vi "sub vi - GET ALL TEMP v6.vi"(0 "LA01-EN":bool, 1 "simulate":bool, 5 "LA02-EN":bool, 7 "LA03-EN":bool, 9 "LA04-EN":bool, 11 "LA05-EN":bool, 12 "Gen Cal Value":dbl) -> (4 "LA01 TEMP":T1, 6 "LA02 TEMP":T1, 8 "LA03 TEMP":T1, 10 "LA04 TEMP":T1, 14 "error":bool, 15 "LA05 TEMP":T1)   [LabVIEW 2013]
uses:
  program files/Global display 4.vi
panel:
  out "LOOP TIME":dbl
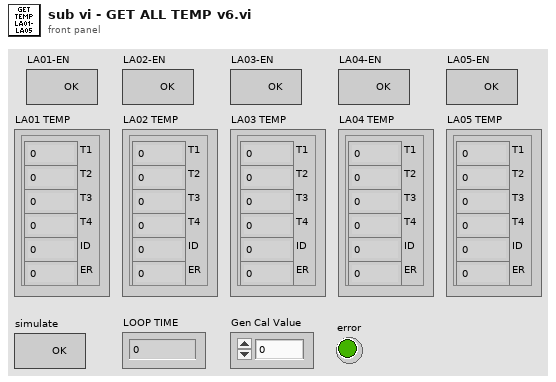
[diagram p1: front panel]
types:
  T1 = cluster{"T1":dbl, "T2":dbl, "T3":dbl, "T4":dbl, "ID":dbl, "ER":dbl}
  T2 = cluster{"1 TL":dbl, "1 TN":dbl, "2 TL":dbl, "2 TN":dbl, "ID":dbl, "ER":dbl}
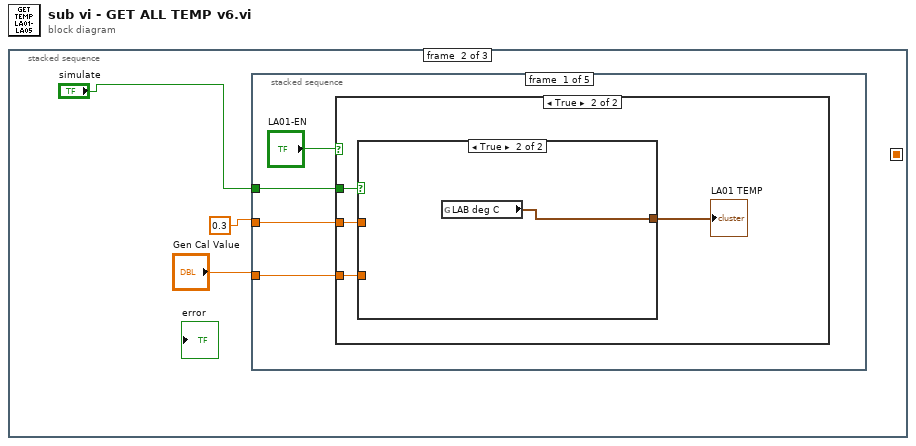
[diagram p0: block diagram]
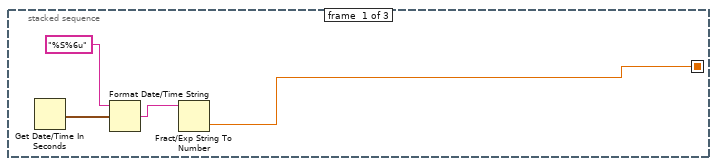
[diagram p2: hidden frame]
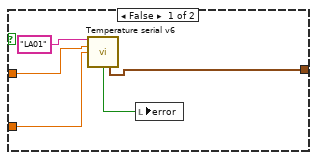
[diagram p4: hidden frame]
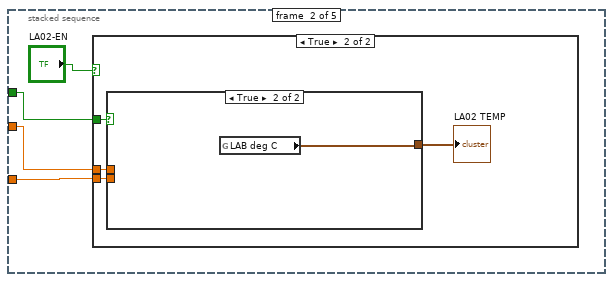
[diagram p5: hidden frame]
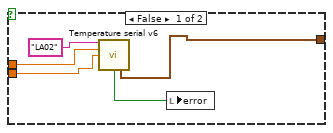
[diagram p7: hidden frame]
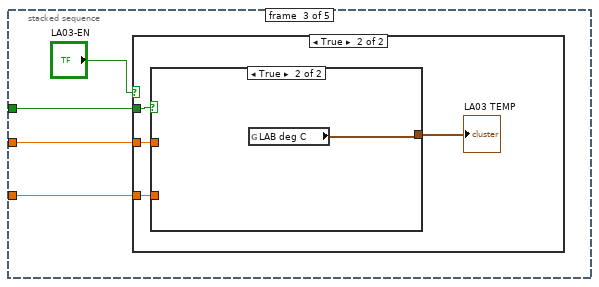
[diagram p8: hidden frame]
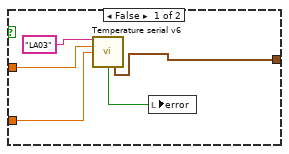
[diagram p10: hidden frame]
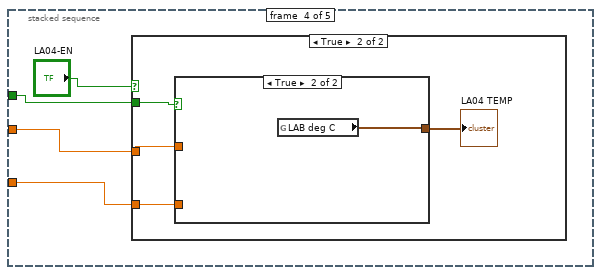
[diagram p11: hidden frame]
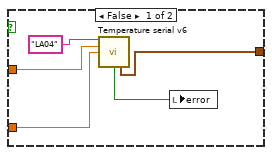
[diagram p13: hidden frame]
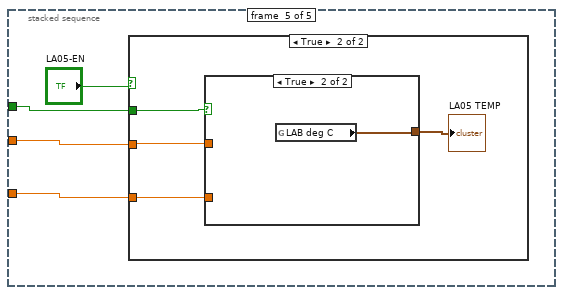
[diagram p14: hidden frame]
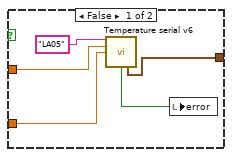
[diagram p16: hidden frame]
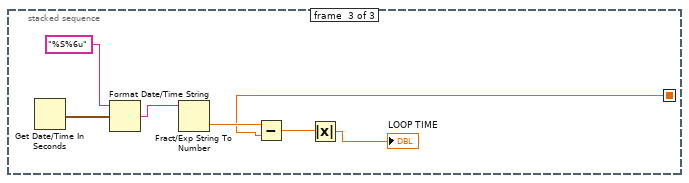
[diagram p17: hidden frame]
diagram:
  n1 = stacked-sequence {
    seq-local: [w1 _ _] -> [_ _ w80]
    frame #0 {
      n2 = Get Date/Time In Seconds() -> (seconds since 1Jan1904=w4:timestamp)
      n3 = Format Date/Time String(time format string (%c)="%S%6u", seconds (now)=w4) -> (date/time string=w2:string)  [unwired: 1 in]
      n4 = Fract/Exp String To Number(string=w2) -> (number=w1:dbl)  [unwired: 3 in, 1 out]
    }
    frame #1 {
      n5 = stacked-sequence {
        tunnel: 0.3 -> [w11 w25 w39 w53 w67]
        tunnel: "Gen Cal Value" -> [w10 w24 w38 w52 w66]
        tunnel: "simulate" -> [w8 w22 w36 w50 w64]
        frame #0 {
          n6 = case shown="True" "LA01-EN" {
            tunnel: w11 -> [_ w15]
            tunnel: w10 -> [_ w14]
            tunnel: w8 -> [_ w12]
            frame False {
            }
            frame True {
              n7 = case shown="True" w12 {
                tunnel: w15 -> [w19 _]
                tunnel: w14 -> [w18 _]
                tunnel: [w16 w21] -> w13
                frame False {
                  n8 = call "Temperature serial v6.vi"("Command String"="LA01", "Time Out (S)"=w19, "CALIB"=w18) -> ("error"=w17:bool, "output cluster"=w16:cluster{dbl, dbl, dbl, dbl, i32, "error #":dbl})  [unwired: 6 in, 5 out]
                  n9 = local write "error"(w17) -> ()
                }
                frame True {
                  n10 = global read "Global display 4.vi" "LAB deg C"() -> (w21:T2)
                }
              }
              "LA01 TEMP" <- w13
            }
          }
        }
        frame #1 {
          n11 = case shown="True" "LA02-EN" {
            tunnel: w25 -> [_ w29]
            tunnel: w24 -> [_ w28]
            tunnel: w22 -> [_ w26]
            frame False {
            }
            frame True {
              n12 = case shown="True" w26 {
                tunnel: w29 -> [w33 _]
                tunnel: w28 -> [w32 _]
                tunnel: [w30 w35] -> w27
                frame False {
                  n13 = call "Temperature serial v6.vi"("Command String"="LA02", "Time Out (S)"=w33, "CALIB"=w32) -> ("error"=w31:bool, "output cluster"=w30:cluster{dbl, dbl, dbl, dbl, i32, "error #":dbl})  [unwired: 6 in, 5 out]
                  n14 = local write "error"(w31) -> ()
                }
                frame True {
                  n15 = global read "Global display 4.vi" "LAB deg C"() -> (w35:T2)
                }
              }
              "LA02 TEMP" <- w27
            }
          }
        }
        frame #2 {
          n16 = case shown="True" "LA03-EN" {
            tunnel: w39 -> [_ w43]
            tunnel: w38 -> [_ w42]
            tunnel: w36 -> [_ w40]
            frame False {
            }
            frame True {
              n17 = case shown="True" w40 {
                tunnel: w43 -> [w47 _]
                tunnel: w42 -> [w46 _]
                tunnel: [w44 w49] -> w41
                frame False {
                  n18 = call "Temperature serial v6.vi"("Command String"="LA03", "Time Out (S)"=w47, "CALIB"=w46) -> ("error"=w45:bool, "output cluster"=w44:cluster{dbl, dbl, dbl, dbl, i32, "error #":dbl})  [unwired: 6 in, 5 out]
                  n19 = local write "error"(w45) -> ()
                }
                frame True {
                  n20 = global read "Global display 4.vi" "LAB deg C"() -> (w49:T2)
                }
              }
              "LA03 TEMP" <- w41
            }
          }
        }
        frame #3 {
          n21 = case shown="True" "LA04-EN" {
            tunnel: w53 -> [_ w57]
            tunnel: w52 -> [_ w56]
            tunnel: w50 -> [_ w54]
            frame False {
            }
            frame True {
              n22 = case shown="True" w54 {
                tunnel: w57 -> [w61 _]
                tunnel: w56 -> [w60 _]
                tunnel: [w58 w63] -> w55
                frame False {
                  n23 = call "Temperature serial v6.vi"("Command String"="LA04", "Time Out (S)"=w61, "CALIB"=w60) -> ("error"=w59:bool, "output cluster"=w58:cluster{dbl, dbl, dbl, dbl, i32, "error #":dbl})  [unwired: 6 in, 5 out]
                  n24 = local write "error"(w59) -> ()
                }
                frame True {
                  n25 = global read "Global display 4.vi" "LAB deg C"() -> (w63:T2)
                }
              }
              "LA04 TEMP" <- w55
            }
          }
        }
        frame #4 {
          n26 = case shown="True" "LA05-EN" {
            tunnel: w67 -> [_ w71]
            tunnel: w66 -> [_ w70]
            tunnel: w64 -> [_ w68]
            frame False {
            }
            frame True {
              n27 = case shown="True" w68 {
                tunnel: w71 -> [w75 _]
                tunnel: w70 -> [w74 _]
                tunnel: [w72 w77] -> w69
                frame False {
                  n28 = call "Temperature serial v6.vi"("Command String"="LA05", "Time Out (S)"=w75, "CALIB"=w74) -> ("error"=w73:bool, "output cluster"=w72:cluster{dbl, dbl, dbl, dbl, i32, "error #":dbl})  [unwired: 6 in, 5 out]
                  n29 = local write "error"(w73) -> ()
                }
                frame True {
                  n30 = global read "Global display 4.vi" "LAB deg C"() -> (w77:T2)
                }
              }
              "LA05 TEMP" <- w69
            }
          }
        }
      }
    }
    frame #2 {
      n31 = Get Date/Time In Seconds() -> (seconds since 1Jan1904=w84:timestamp)
      n32 = Format Date/Time String(time format string (%c)="%S%6u", seconds (now)=w84) -> (date/time string=w82:string)  [unwired: 1 in]
      n33 = Fract/Exp String To Number(string=w82) -> (number=w81:dbl)  [unwired: 3 in, 1 out]
      n34 = Subtract(x=w81, y=w80) -> (x-y=w79:dbl)
      n35 = Absolute Value(x=w79) -> (abs(x)=→"LOOP TIME":dbl)
    }
  }
